vi "database_connection_write_dev_MQTT.vi"(5 "ODBC data source name":string="amrc_monitoring", 6 "error in (no error)":errorcluster, 7 "G1?":u32, 8 "current time":timestamp, 9 "data 2":dbl[](array[numeric]), 10 "Machine Data":T4={"Zload"="", "Yload"="", "Xload"="", "path_position"="", "Fovr"="", "SspeedOvr"="", "Program Name"="", "Program status"="", "Block of code being executed"="", "Line of code"="", "Machine availability"="", "Emergency status"="", "Controller mode"="", "Tool_id"="UNAVAILABLE"}, 11 "Machine type":string) -> (3 "error out":errorcluster)   [LabVIEW 2017]
uses:
  mqtt Folder/src/class/mqtt/mqttTypedef/mqttConnectionStatus.ctl
  mqtt Folder/src/class/mqtt/mqttTypedef/mqttConnectionMeta.ctl
  mqtt Folder/src/class/mqtt/mqttTypedef/mqttQOSlevel.ctl
  mqtt Folder/src/class/mqtt/mqttConfigFunction.ctl
  mqtt Folder/src/class/mqtt/mqttTypedef/mqttBroker.ctl
  mqtt Folder/src/class/mqtt/mqttTypedef/mqttConnectionFlags.ctl
  mqtt Folder/src/class/mqtt/mqttTypedef/mqttWillInformation.ctl
  mqtt Folder/src/class/mqtt/mqttTXqueue/mqttTXdataQueueFunction.ctl
  mqtt Folder/src/class/mqtt/mqttTXqueue/mqttRXsubscriptionEventFunction.ctl
  <vilib>/addons/database/Connection.llb/DB Tools Open Connec (Path).vi
  <vilib>/addons/database/Connection.llb/Conn Execute.vi
  <vilib>/addons/database/Recordset.llb/Rec Destroy - Connection.vi
  <vilib>/regexp/Match Regular Expression.xnode
  <vilib>/addons/database/NI_Database_API.lvlib
  mqtt Folder/src/class/mqtt/mqtt.lvclass
panel:
  out "error out 3":errorcluster
  out "publishSuccess 2":bool=TRUE
  out "publishMessageID 2":u16 format="%02x"
  out "valueSent 2":string="14:19:17.238_"
  in  "connMeta 2":T1
  in  "topic 2":string="a/b"
  out "connStatus 2":T3
  out "sessionPresent 2":bool
  out "string":string="(timestamp,machine_status,g1,tool_id,force_acc_raw_data,spike_raw_data,spindle_load,spindle_speed,feed_rate,I,J,K,X,Y,Z,position_A,position_B ,Xload,Yload,Zload,Aload,Bload,program_number,accel_x_rms,accel_y_rms,accel_z_rms,force_x_rms,force_y_rms,force_z_rms,axial_force_rms, torque_rms,bending_x_rms,bending_y_rms,estop,block_code,fovr,sspeedovr,program_name,line) VALUES ("
  out "data 3":dbl[](array[numeric])
  out "path_position":string
  out "x = y?":bool
  out "submatch 1":string
  out "after match 3":string
  out "empty? 2":bool
  out "after match 2":string
  out "resulting string 4":string
  out "Xload":string
  out "concatenated string 6":string
  out "resulting string 3":string
  out "concatenated string 2":string
  out "resulting string 2":string
  out "ODBC data source name 2":string="amrc_monitoring"
  out "resulting string":string
  out "size(s)":i32
  out "concatenated string 5":string
  out "concatenated string 3":string
  out "concatenated string":string
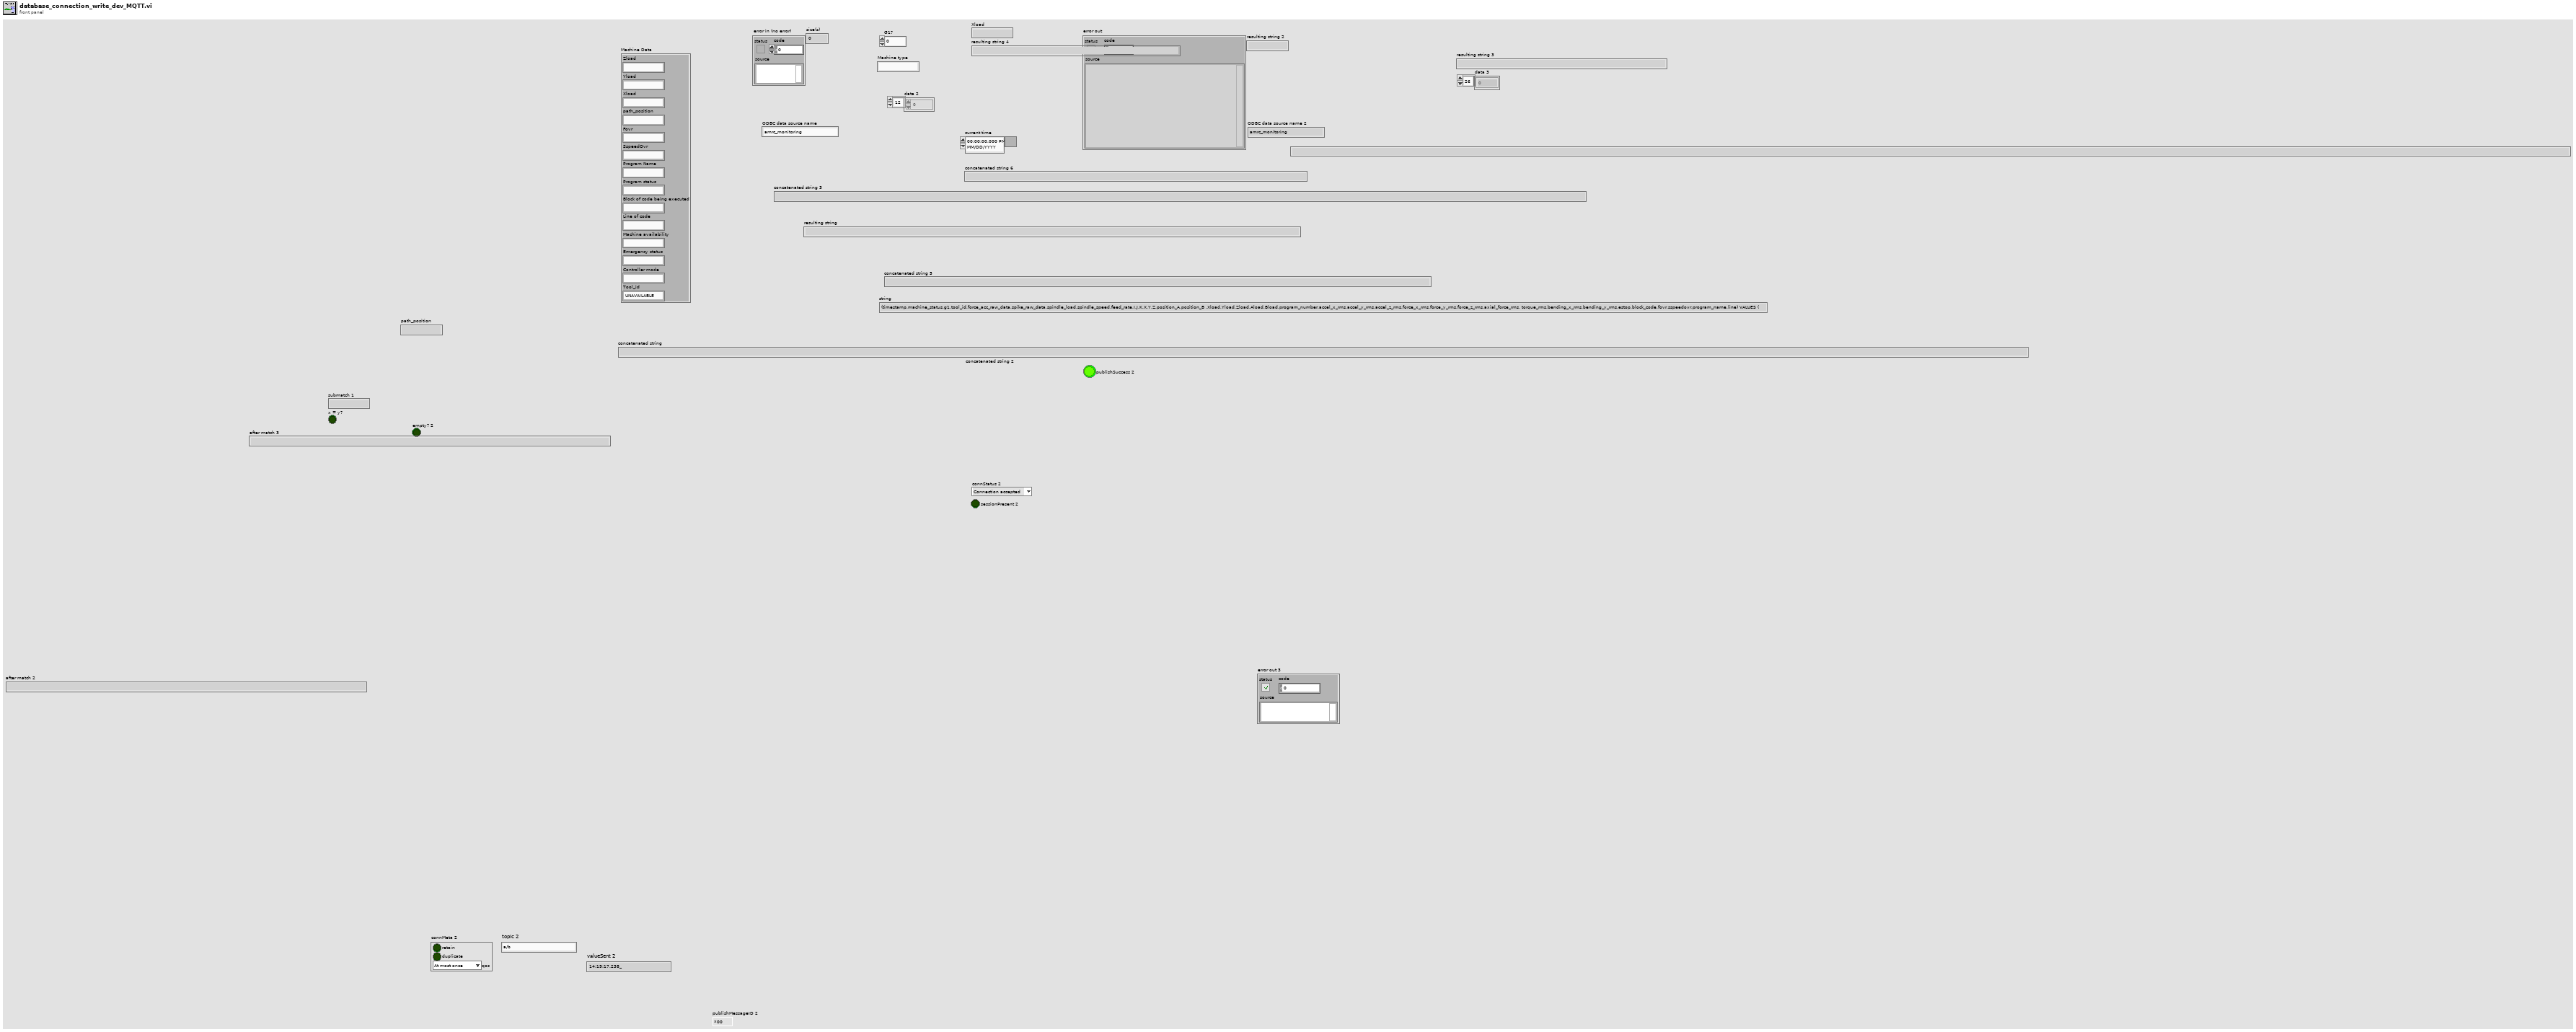
[diagram p1: front panel]
types:
  T1 = typedef "mqttConnectionMeta.ctl" = cluster{"retain":bool, "duplicate":bool, "qos":T2}
  T2 = typedef "mqttQOSlevel.ctl" = enum8{"At most once", "At least once", "Exactly once", "Reserved"}
  T3 = typedef "mqttConnectionStatus.ctl" = enum16{"Connection accepted", "Connection refused: unacceptable protocol version", "Connection refused: identifier rejected", "Connection refused: Server unavailable", "Connection refused: bad user name or password", "Connection refused: not authorized"}
  T4 = cluster{"Zload":string, "Yload":string, "Xload":string, "path_position":string, "Fovr":string, "SspeedOvr":string, "Program Name":string, "Program status":string, "Block of code being executed":string, "Line of code":string, "Machine availability":string, "Emergency status":string, "Controller mode":string, "Tool_id":string}
  T5 = typedef "mqttRXsubscriptionEventFunction.ctl" = enum16{"init", "deinit", "getEventRef", "event"}
  T6 = typedef "mqttTXdataQueueFunction.ctl" = enum16{"init", "deinit", "getQueue", "enqueue"}
  T7 = typedef "mqttWillInformation.ctl" = cluster{"User Name":string, "Password":string}
  T8 = typedef "mqttConnectionFlags.ctl" = cluster{"reserved":bool, "clean session":bool, "will flag":bool, "willQOS":enum8{"At most once", "At least once", "Exactly once", "Reserved"}, "will retain":bool, "password":bool, "user name":bool}
  T9 = typedef "mqttBroker.ctl" = cluster{"address":string, "port":u16, "connTimeout":i32, "writeTimeout":i32, "readTimeout":i32, "subTimeout":i32}
  T10 = typedef "mqtt.lvclass/mqttConfigFunction.ctl" = enum16{"init", "deinit", "set", "get"}
  T11 = enum8{"Enabled", "Disabled", "Disabled and Grayed Out"}
  T12 = typedef "NI_Database_API.lvlib/Conn ObjectReference.ctl" = refnum<k1>
  T13 = typedef "NI_Database_API.lvlib/Rec ObjectReference.ctl" = refnum<k1>
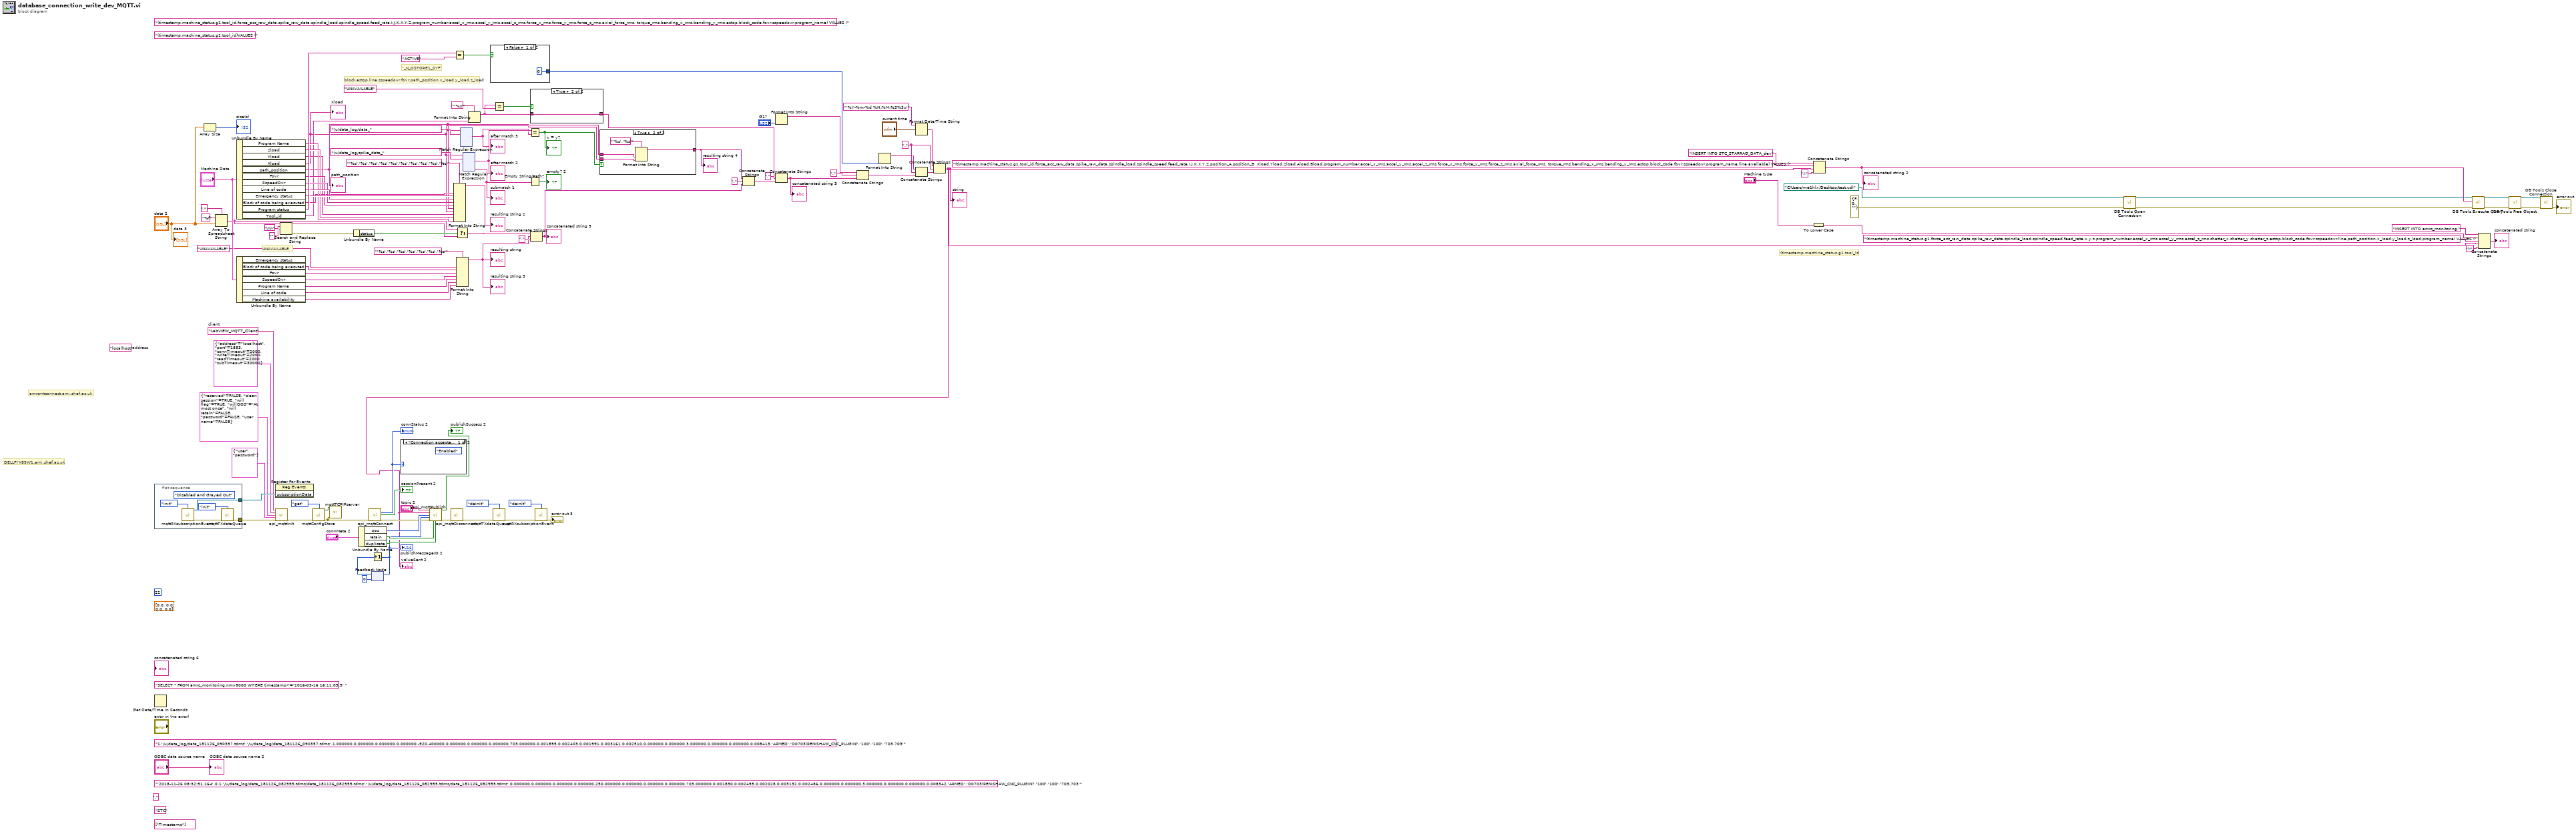
[diagram p0: block diagram]
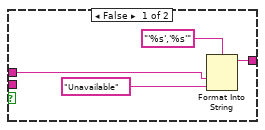
[diagram p3: hidden frame]
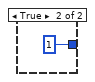
[diagram p5: hidden frame]
diagram:
  (unwired) "localhost"  # address
  w24 = "LabVIEW_MQTT_Client"  # client
  (unwired) "(timestamp,machine_status,g1,tool_id,force_acc_raw_data,spike_raw_data,spindle_load,spindle_speed,feed_rate,I,J,K,X,Y,Z,program_number,accel_x_rms,accel_y_rms,accel_z_rms,force_x_rms,force_y_rms,force_z_rms,axial_force_rms, torque_rms,bending_x_rms,bending_y_rms,estop,block_code,fovr,sspeedovr,program_name) VALUES (" ("string")
  (unwired) "(timestamp,machine_status,g1,tool_id)VALUES (" ("string")
  (unwired) dbl[] [0.0, 0.0, 0.0, 0.0]
  (unwired) "1,'/u/data_log/data_181126_090357.tdms','/u/data_log/data_181126_090357.tdms',1.000000,0.000000,0.000000,0.000000,-920.400000,0.000000,0.000000,0.000000,703.000000,0.001895,0.002403,0.001991,0.003161,0.002510,0.000000,0.000000,3.000000,0.000000,0.000000,0.008413,'ARMED','O0703(RENISHAW_CNC_PLUGIN)','100','100','703.703'" ("concatenated string 4")
  (unwired) "'2018-11-26 08:32:51.164',0,1,'/u/data_log/data_181126_082955.tdms/data_181126_082955.tdms','/u/data_log/data_181126_082955.tdms/data_181126_082955.tdms',0.000000,0.000000,0.000000,0.000000,250.000000,0.000000,0.000000,0.000000,703.000000,0.001830,0.002455,0.002028,0.003132,0.002486,0.000000,0.000000,3.000000,0.000000,0.000000,0.008342,'ARMED','O0703(RENISHAW_CNC_PLUGIN)','100','100','703.703'" ("concatenated string 2")
  (unwired) 22
  (unwired) "," ("string")
  (unwired) string[] ["Timestamp"]
  (unwired) "STC"
  w75 = "," ("string")
  (unwired) "SELECT * FROM amrc_monitoring.nmv8000 WHERE timestamp>='2016-03-16 16:11:05.5' " ("SQL query")
  # "amrcmtconnect.ami.shef.ac.uk"
  # "DELLFYX89W1.ami.shef.ac.uk"
  # "(timestamp,machine_status,g1,tool_id"
  # "'_N_OSTORE1_SYF'"
  # "UNAVAILABLE"
  # "block,estop,line,sspeedovr,fovr,path_position,x_load,y_load,z_load"
  n1 = flat-sequence {
    tunnel: [w120] -> w29
    tunnel: [w117] -> w25
    frame #0 {
      (unwired) T11."Disabled and Grayed Out" ("Disabled")
      n2 = call "mqttRXsubscriptionEvent.vi"("function"=mqttRXsubscriptionEventFunction."init") -> ("subscriptionData"=w117:refnum<user-event>, "error out"=w119:errorcluster)  [unwired: 13 in]
      n3 = call "mqttTXdataQueue.vi"("function"=mqttTXdataQueueFunction."init", "error in (no error)"=w119) -> ("error out"=w120:errorcluster)  [unwired: 12 in, 1 out]
    }
  }
  n4 = Get Date/Time In Seconds() -> ()  [unwired: 1 out]
  n5 = Array Size(array="data 2") -> (size(s)=→"size(s)":i32)
  n6 = Array To Spreadsheet String(delimiter (Tab)=",", array="data 2", 3:"%f" ("format string")) -> (spreadsheet string=w101:string)
  n7 = Unbundle By Name("Machine Data") -> ("Program Name"=w88:string, "Zload"=w92:string, "Yload"=w53:string, "Xload"=w34:string, "path_position"=w35:string, "Fovr"=w93:string, "SspeedOvr"=w94:string, "Line of code"=w95:string, "Emergency status"=w96:string, "Block of code being executed"=w86:string, "Program status"=w114:string, "Tool_id"=w80:string)
  "Xload" <- w34
  "path_position" <- w35
  n8 = Unbundle By Name("Machine Data") -> ("Block of code being executed"=w60:string, "Fovr"=w59:string, "SspeedOvr"=w58:string, "Program Name"=w57:string, "Line of code"=w32:string, "Machine availability"=w30:string)  [unwired: 1 out]
  n9 = register-events(w25) -> ()  [unwired: 2 in, 2 out]
  n10 = call "api_mqttInit.vi"("client"=w24, "broker"=T9 {"address"="localhost", "port"=1883, "connTimeout"=2000, "writeTimeout"=2000, "readTimeout"=2000, "subTimeout"=30000}, "connFlags"=T8 {"reserved"=FALSE, "clean session"=TRUE, "will flag"=TRUE, "willQOS"=enum."At most once", "will retain"=FALSE, "password"=FALSE, "user name"=FALSE}, "User Info"=T7 {"User Name"="User", "Password"="password"}, "error in (no error)"=w29) -> ("error out"=w27:errorcluster)  [unwired: 10 in]
  n11 = Search and Replace String(input string=w101, search string="\r\n", replace string="" ("replace string (\"\")")) -> (result string=w102:string, error out=w104:errorcluster)  [unwired: 5 in, 2 out]
  n12 = call "mqttConfigStore.vi"("function"=mqttConfigFunction."get", "error in (no error)"=w27) -> ("mqtt.lvclass out"=w26:refnum<class "mqtt.lvclass">, "error out"=w18:errorcluster)  [unwired: 12 in]
  n13 = call "mqttTCPIPserver.vi"("mqtt.lvclass"=w26, "error in (no error)"=w18) -> ()  [unwired: 12 in, 2 out]
  n14 = Unbundle By Name(w104) -> ("status"=w103:bool)
  n15 = Unbundle By Name("connMeta 2") -> ("qos"=w15:T2, "retain"=w14:bool, "duplicate"=w13:bool)
  n16 = call "api_mqttConnect.vi"("error in (no error)"=w18) -> ("connStatus"=w20:T3, "sessionPresent"=→"sessionPresent 2":bool, "error out"=w12:errorcluster)  [unwired: 11 in, 1 out]
  "connStatus 2" <- w20
  n17 = feedback #1(u16 0) -> (w10:u16)
  n18 = Increment(x=w10) -> (x+1=w9:u16)
  "publishMessageID 2" <- w9
  n19 = feedback-in #1(w9) -> ()
  n20 = case shown="\"Connection accepted\"" w20 {
    frame "Connection accepted" {
      (unwired) T11."Enabled" ("Disabled")
    }
    frame Default {
    }
  }
  n21 = Format Into String(format string="'%s','%s','%s','%s','%s','%s','%s','%s','%s','%s'", w86, w96, w95, w94, w93, w35, w34, w53, w92, w88) -> (resulting string=→"resulting string 2":string)  [unwired: 2 in, 1 out]
  n22 = Equal?(x=w114, y="ACTIVE") -> (x = y?=w112:bool)
  n23 = Select(t=w101, s=w103, f=w102) -> (s? t:f=w89:string)
  n24 = Format Into String(format string="'%s','%s','%s','%s','%s','%s','%s'", "UNAVAILABLE" ("format string"), w60, w59, w58, w57, w32, w30) -> (resulting string=w52:string)  [unwired: 2 in, 1 out]
  "resulting string" <- w52
  "resulting string 3" <- w52
  n25 = xnode "Match Regular Expression"("input string"=w35, "regular expression"="/u/data_log/data_") -> ("after match"=w37:string)  [unwired: 4 in, 5 out]
  "after match 3" <- w37
  n26 = xnode "Match Regular Expression"("input string"=w34, "regular expression"="/u/data_log/spike_data_") -> ("after match"=w38:string, "submatch 1"=w39:string)  [unwired: 4 in, 4 out]
  "after match 2" <- w38
  "submatch 1" <- w39
  n27 = Format Into String(format string="'%s'", w80) -> (resulting string=w79:string)  [unwired: 2 in, 1 out]
  n28 = case shown="False" w112 {
    tunnel: [0 1] -> w49
    frame False {
    }
    frame True {
    }
  }
  n29 = Equal?(x=w79, y="UNAVAILABLE") -> (x = y?=w111:bool)
  n30 = Equal?(x=w38, y=w37) -> (x = y?=w36:bool)
  "x = y?" <- w36
  n31 = Empty String/Path?(string/path=w39) -> (empty?=→"empty? 2":bool)
  n32 = case shown="True" w111 {
    tunnel: w79 -> [w124 w125]
    tunnel: [w124 w125] -> w31
    frame False {
    }
    frame True {
    }
  }
  n33 = Concatenate Strings(w89, "," ("string"), w52) -> (w46:string)
  "concatenated string 5" <- w46
  n34 = case shown="True" w36 {
    tunnel: w35 -> [w128 w130]
    tunnel: w34 -> [_ w133]
    tunnel: [w127 w131] -> w33
    frame False {
      n35 = Format Into String(format string="'%s','%s'", w128, "Unavailable" ("Tool_id")) -> (resulting string=w127:string)  [unwired: 2 in, 1 out]
    }
    frame True {
      n36 = Format Into String(format string="'%s','%s'", w130, w133) -> (resulting string=w131:string)  [unwired: 2 in, 1 out]
    }
  }
  "resulting string 4" <- w33
  n37 = Concatenate Strings(w33, "," ("string"), w46) -> (w44:string)
  n38 = Format Into String("G1?") -> (resulting string=w73:string)  [unwired: 3 in, 1 out]
  n39 = Concatenate Strings(w31, "," ("string"), w44) -> (w50:string)
  "concatenated string 3" <- w50
  n40 = Concatenate Strings(w73, "," ("string"), w50) -> (w51:string)
  n41 = Format Into String(w49) -> (resulting string=w74:string)  [unwired: 3 in, 1 out]
  n42 = Format Date/Time String(time format string (%c)="'%Y-%m-%d %H:%M:%S%3u'", seconds (now)="current time") -> (date/time string=w76:string)  [unwired: 1 in]
  n43 = Concatenate Strings(w74, w75, w51) -> (w107:string)
  n44 = Concatenate Strings(w76, w75, w107) -> (w1:string)
  "string" <- w1
  "valueSent 2" <- w1
  n45 = call "api_mqttPublish.vi"("topic"="topic 2", "value"=w1, "QoS (At most once)"=w15, "messageID"=w9, "error in (no error)"=w12, "retain(F)"=w14, "duplicate(F)"=w13) -> ("success"=→"publishSuccess 2":bool, "error out"=w2:errorcluster)  [unwired: 7 in]
  n46 = call "api_mqttDisconnect.vi"("error in (no error)"=w2) -> ("error out"=w6:errorcluster)  [unwired: 13 in, 1 out]
  n47 = call "mqttTXdataQueue.vi"("function"=mqttTXdataQueueFunction."deinit", "error in (no error)"=w6) -> ("error out"=w4:errorcluster)  [unwired: 12 in, 1 out]
  n48 = call "mqttRXsubscriptionEvent.vi"("function"=mqttRXsubscriptionEventFunction."deinit", "error in (no error)"=w4) -> ("error out"=→"error out 3":errorcluster)  [unwired: 12 in, 1 out]
  n49 = To Lower Case(string="Machine type") -> (all lower case string=w98:string)
  n50 = Concatenate Strings("INSERT INTO STC_STARRAG_DATA_dev" ("string"), "(timestamp,machine_status,g1,tool_id,force_acc_raw_data,spike_raw_data,spindle_load,spindle_speed,feed_rate,I,J,K,X,Y,Z,position_A,position_B ,Xload,Yload,Zload,Aload,Bload,program_number,accel_x_rms,accel_y_rms,accel_z_rms,force_x_rms,force_y_rms,force_z_rms,axial_force_rms, torque_rms,bending_x_rms,bending_y_rms,estop,block_code,fovr,sspeedovr,program_name,line,available) VALUES (" ("string"), w1, ");" ("string")) -> (w72:string)
  "concatenated string 2" <- w72
  n51 = call-poly <vilib>:"DB Tools Open Connection.vi"("error in (no error)"=errorcluster {"status"=FALSE, "code"=0, "source"=""}, "connection information"=path "C:/Users/me1hlx/Desktop/test.udl") -> ("error out"=w71:errorcluster, "connection reference"=w65:T12)  [unwired: 6 in]
  n52 = call-poly <vilib>:"DB Tools Execute Query.vi"("error in (no error)"=w71, "SQL query"=w72, "connection reference"=w65) -> ("error out"=w68:errorcluster, "recordset reference"=w69:T13)  [unwired: 5 in]
  n53 = Concatenate Strings("INSERT INTO amrc_monitoring." ("string"), w98, "(timestamp,machine_status,g1,force_acc_raw_data,spike_raw_data,spindle_load,spindle_speed,feed_rate,x,y,z,program_number,accel_x_rms,accel_y_rms,accel_z_rms,chatter_x,chatter_y,chatter_z,estop,block_code,fovr,sspeedovr,line,path_position,x_load,y_load,z_load,program_name) VALUES (" ("string"), w1, ");" ("string")) -> (→"concatenated string":string)
  n54 = call-poly <vilib>:"DB Tools Free Object.vi"("error in (no error)"=w68, "recordset reference"=w69) -> ("error out"=w66:errorcluster, "connection reference"=w67:T12)  [unwired: 8 in]
  n55 = call <vilib>:"DB Tools Close Connection.vi"("error in (no error)"=w66, "connection reference"=w67) -> ("error out"=→"error out":errorcluster)  [unwired: 5 in]
  "ODBC data source name 2" <- "ODBC data source name"
  "data 3" <- "data 2"
